vi "Moving_Point_Average.vi"(10 "Averaging Points":i32, 11 "X":dbl[](array[numeric])) -> (2 "Moving Average of X":dbl[](array[numeric]))   [LabVIEW 2011]
uses:
  <vilib>/ptbypt/NI_PtbyPt.lvlib
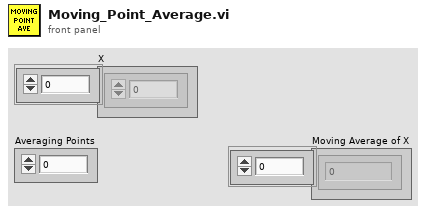
[diagram p1: front panel]
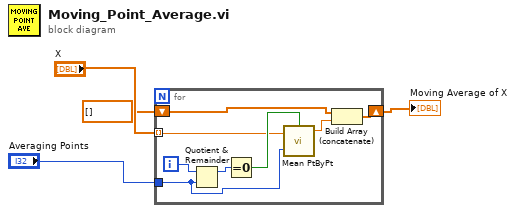
[diagram p0: block diagram]
diagram:
  n1 = for {
    tunnel: "X" -> [w9] mode=indexing
    shift-right: [w7] -> w4
    shift-left: dbl[] [] -> [w6]
    tunnel: "Averaging Points" -> [w5]
    i -> [w12]
    n2 = Quotient & Remainder(x=w12, y=w5) -> (x-y*floor(x/y)=w11:i32)  [unwired: 1 out]
    n3 = Equal To 0?(x=w11) -> (x = 0?=w10:bool)
    n4 = call <vilib>:"Mean PtByPt.vi"("x"=w9, "sample length"=w5, "initialize"=w10) -> ("mean"=w8:dbl)  [unwired: 1 in, 1 out]
    n5 = Build Array (concatenate)(w6, w8) -> (w7:dbl[])
  }
  "Moving Average of X" <- w4
